vi "Get Transfer Configurations.vi"(11 "Transfer Group Configuration in":refnum<class "Transfer Group Configuration.lvclass">) -> (2 "Transfer Configurations":refnum<class "Transfer Configuration.lvclass">[](array[class]), 3 "Transfer Group Configuration out":refnum<class "Transfer Group Configuration.lvclass">)   [LabVIEW 2017, in "Data Sharing Framework Engine.lvlib" / "Transfer Group Configuration.lvclass"]
uses:
  Transfer Group Configuration.lvclass
  Source/Data Sharing Framework Core/Engine/Transfer Configuration/Transfer Configuration.lvclass
  Transfer Group Configuration.lvclass/Transfer Group Configuration.ctl
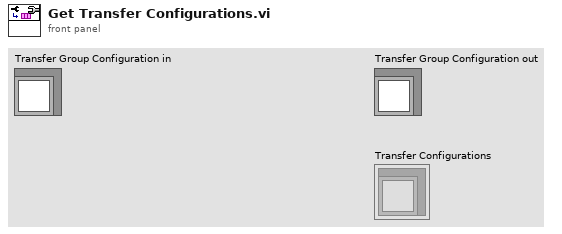
[diagram p1: front panel]
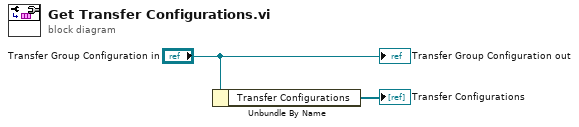
[diagram p0: block diagram]
diagram:
  n1 = Unbundle By Name("Transfer Group Configuration in") -> ("Transfer Configurations"=→"Transfer Configurations":refnum<class "Transfer Configuration.lvclass">[])
  "Transfer Group Configuration out" <- "Transfer Group Configuration in"
